vi "Test.vi"() -> ()   [LabVIEW 2020]
panel:
  out "concatenated string":string
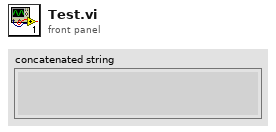
[diagram p1: front panel]
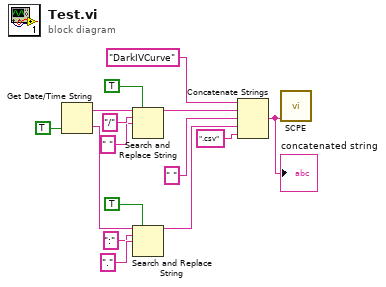
[diagram p0: block diagram]
diagram:
  n1 = Get Date/Time String(want seconds? (F)=TRUE) -> (date string=w13:string, time string=w5:string)  [unwired: 2 in]
  n2 = Search and Replace String(replace all?=TRUE ("replace all? (F)"), input string=w13, search string="/" ("substring (\"\")"), replace string=" " ("replace string (\"\")")) -> (result string=w9:string)  [unwired: 4 in, 3 out]
  n3 = Search and Replace String(replace all?=TRUE ("replace all? (F)"), input string=w5, search string=":" ("substring (\"\")"), replace string="." ("replace string (\"\")")) -> (result string=w2:string)  [unwired: 4 in, 3 out]
  n4 = Concatenate Strings("DarkIVCurve" ("string"), w9, " " ("string"), w2, ".csv" ("string")) -> (w15:string)
  "concatenated string" <- w15
  n5 = call "SCPE.vi"("FileName"=w15) -> ()  [unwired: 4 in, 6 out]
